vi "turtlesimtest.vi"   [LabVIEW 2014]
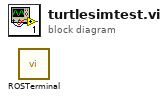
[diagram p0: block diagram]
diagram:
  n1 = call <vilib>:"ROSTerminal.vi"() -> ()  [unwired: 2 in]
